vi "RGBA To ARGB.vi"(10 "Depth":u32, 11 "RGBA":u8[](array[numeric])) -> (3 "ARGB":u8[](array[numeric]))   [LabVIEW 2020, in "G-Image.lvlib"]
doc: "Convert the image memory layout from RGBA to (A)RGB. Applies to 24-bit and 32-bit images."
uses:
  G-Image.lvlib
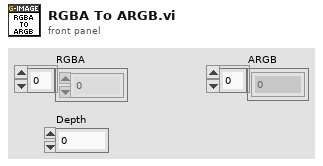
[diagram p1: front panel]
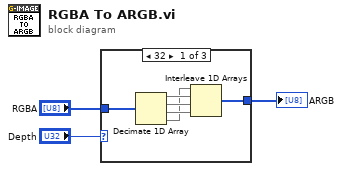
[diagram p0: block diagram]
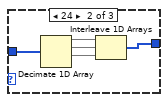
[diagram p2: hidden frame]
diagram:
  n1 = case shown="32" "Depth" {
    tunnel: "RGBA" -> [w9 w14 w15]
    tunnel: [w8 w13 w15] -> w1
    frame 32 {
      n2 = Decimate 1D Array(w9) -> (w7:u8[], w6:u8[], w5:u8[], w4:u8[])
      n3 = Interleave 1D Arrays(w4, w7, w6, w5) -> (w8:u8[])
    }
    frame 24 {
      n4 = Decimate 1D Array(w14) -> (w12:u8[], w11:u8[], w10:u8[])  [unwired: 1 out]
      n5 = Interleave 1D Arrays(w12, w11, w10) -> (w13:u8[])
    }
    frame Default {
      # "1, 2, 4, 8"
    }
  }
  "ARGB" <- w1
